vi "OpenVIs.vi"(8 "error in (no error)":errorcluster, 9 "Title Prefix In":string, 10 "VI Screenshots":T1, 11 "VI Path":path) -> (0 "error out":errorcluster, 2 "VI Screenshots out":T1)   [LabVIEW 2015, in "VIDiffUtilities.lvlib"]
uses:
  VIDiffUtilities.lvlib
  Screenshots/VIScreenshots.ctl
  Screenshots/ScreenshotInfo.ctl
  Screenshots/Screenshot Type.ctl
  FilePaths.ctl
  Screenshots/VIDiffScreenshots.lvlib
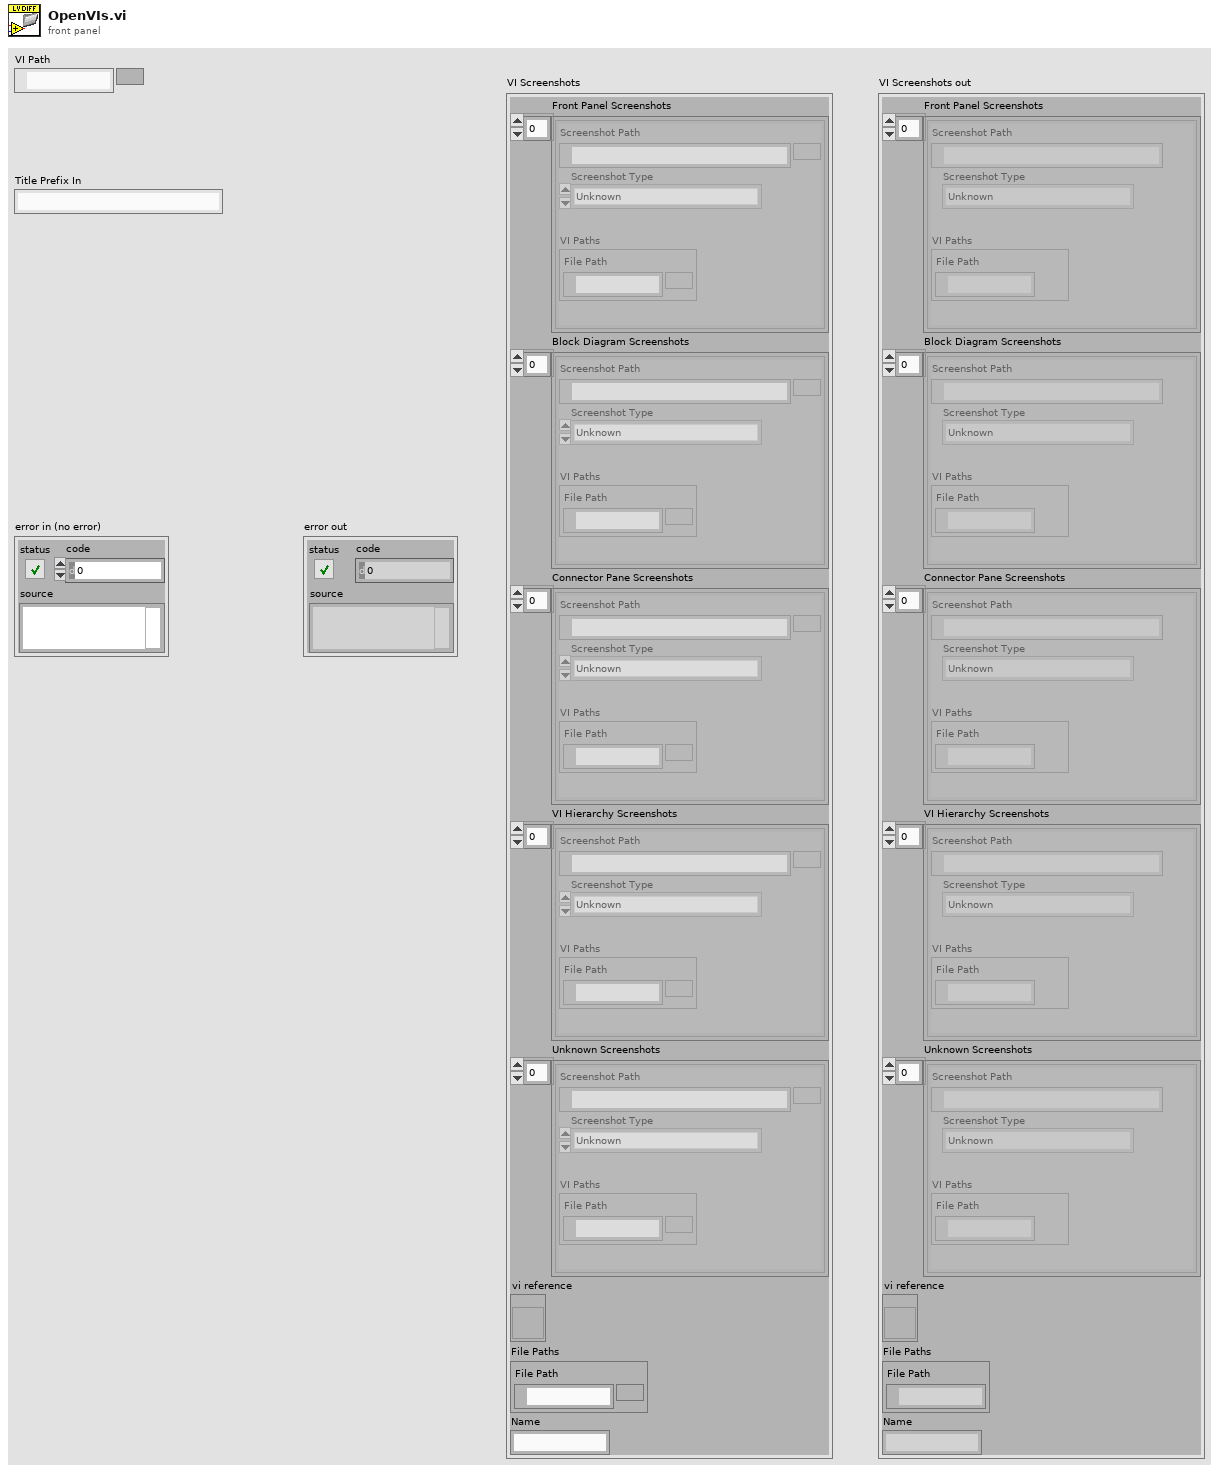
[diagram p1: front panel]
types:
  T1 = typedef "VIDiffScreenshots.lvlib/VIScreenshots.ctl" = cluster{"Front Panel Screenshots":T2[], "Block Diagram Screenshots":T2[], "Connector Pane Screenshots":T2[], "VI Hierarchy Screenshots":T2[], "Unknown Screenshots":T2[], "vi reference":refnum<vi>, "File Paths":cluster{"File Path":path}, "Name":string}
  T2 = typedef "VIDiffScreenshots.lvlib/ScreenshotInfo.ctl" = cluster{"Screenshot Path":path, "Screenshot Type":T3, "VI Paths":T4}
  T3 = typedef "VIDiffScreenshots.lvlib/Screenshot Type.ctl" = enum16{"Unknown", "Front Panel", "Connector Pane", "Block Diagram", "VI Hierarchy"}
  T4 = typedef "VIDiffUtilities.lvlib/FilePaths.ctl" = cluster{"File Path":path}
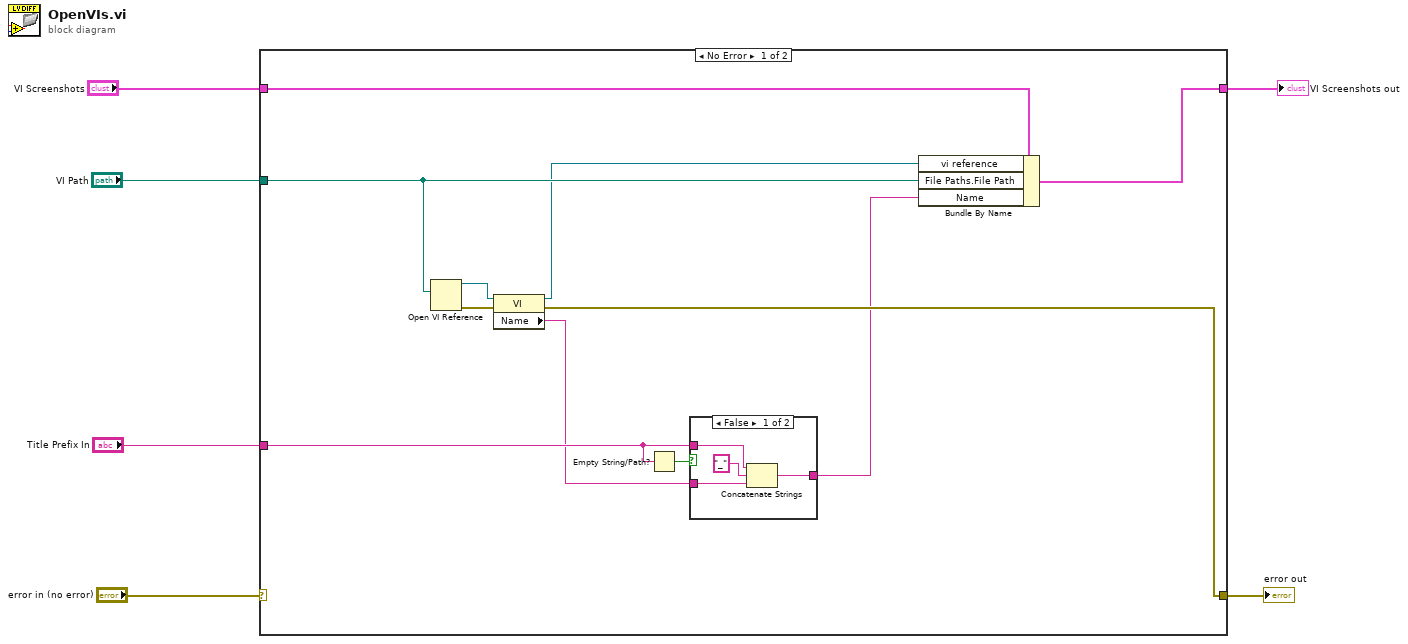
[diagram p0: block diagram]
diagram:
  n1 = case shown="No Error" "error in (no error)" {
    selector: "error in (no error)" -> [_ w24]
    tunnel: [w12 w24] -> w5
    tunnel: "VI Screenshots" -> [w17 w23]
    tunnel: [w16 w23] -> w3
    tunnel: "VI Path" -> [w15 _]
    tunnel: "Title Prefix In" -> [w9 _]
    frame No Error {
      n2 = Open VI Reference(vi path=w15) -> (vi reference=w14:refnum<vi>, error out=w13:errorcluster)  [unwired: 5 in]
      n3 = property class="VI"(reference=w14, error in=w13) -> (reference out=w11:refnum<vi>, error out=w12:errorcluster, "Name"=w8:string)
      n4 = Empty String/Path?(string/path=w9) -> (empty?=w10:bool)
      n5 = case shown="False" w10 {
        tunnel: w8 -> [w21 w22]
        tunnel: [w20 w22] -> w7
        tunnel: w9 -> [w18 _]
        frame False {
          n6 = Concatenate Strings(w18, "_" ("string"), w21) -> (w20:string)
        }
        frame True {
        }
      }
      n7 = Bundle By Name(cluster=w17, "vi reference"=w11, "File Paths.File Path"=w15, "Name"=w7) -> (w16:T1)
    }
    frame Error {
    }
  }
  "error out" <- w5
  "VI Screenshots out" <- w3
